vi "axisParameters.vi"(4 "colOffset":i32, 5 "rowOffset":i32, 6 "cols":i32, 7 "rows":i32, 8 "pixelSize":dbl=3e-05 format="%#_6pm", 9 "plotUnitsPrefix":dbl=1000.0) -> (0 "yAxisScaled":dbl[](array[numeric]), 1 "xAxisScaled":dbl[](array[numeric]), 2 "yAxis":dbl[](array[numeric]), 3 "xAxis":dbl[](array[numeric]))   [LabVIEW 2021]
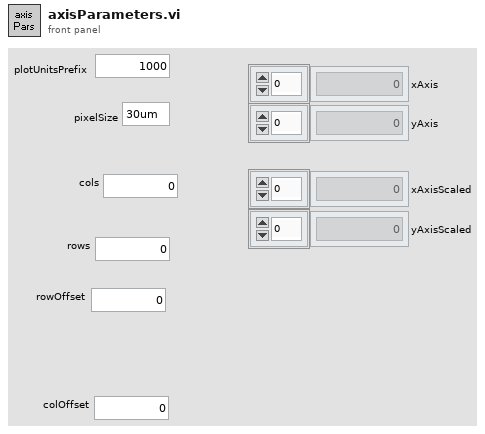
[diagram p1: front panel]
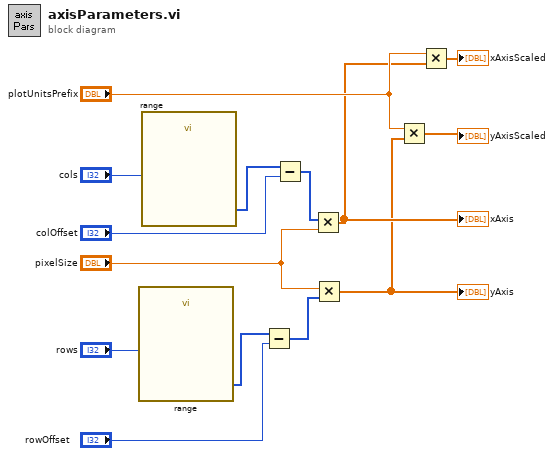
[diagram p0: block diagram]
diagram:
  n1 = call "range.vi"("end"="rows") -> ("range"=w13:i32[])  [unwired: 10 in]
  n2 = call "range.vi"("end"="cols") -> ("range"=w14:i32[])  [unwired: 10 in]
  n3 = Subtract(x=w13, y="rowOffset") -> (x-y=w10:i32[])
  n4 = Subtract(x=w14, y="colOffset") -> (x-y=w11:i32[])
  n5 = Multiply(x=w11, y="pixelSize") -> (x*y=w4:dbl[])
  "xAxis" <- w4
  n6 = Multiply(x="pixelSize", y=w10) -> (x*y=w3:dbl[])
  "yAxis" <- w3
  n7 = Multiply(x="plotUnitsPrefix", y=w3) -> (x*y=→"yAxisScaled":dbl[])
  n8 = Multiply(x="plotUnitsPrefix", y=w4) -> (x*y=→"xAxisScaled":dbl[])
